vi "Get Date Yields.vi"(8 "error in (no error)":errorcluster, 11 "Programing Logic in":refnum<class "Programing Logic.lvclass">) -> (0 "error out":errorcluster, 2 "Cluster":T1, 3 "Programing Logic out":refnum<class "Programing Logic.lvclass">)   [LabVIEW 2014, in "Programing Logic.lvclass"]
uses:
  Programming Logic/Programing Logic.lvclass
  Programming Logic/Programing Logic.lvclass/Programing Logic.ctl
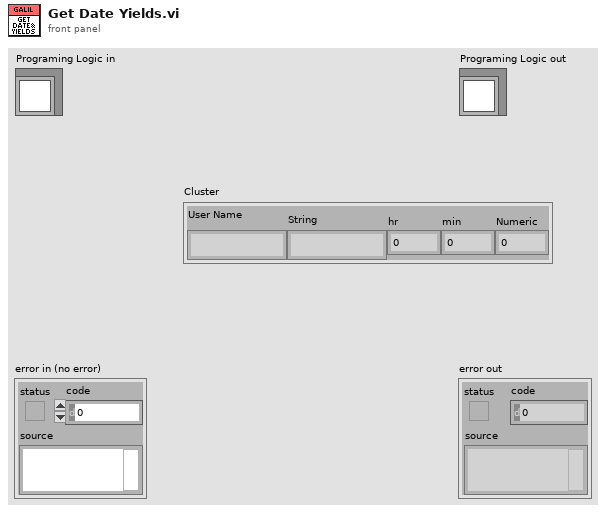
[diagram p1: front panel]
types:
  T1 = cluster{"User Name":string, "String":string, "Numeric":dbl, "min":dbl, "hr":dbl}
  T2 = cluster{"User":string, "Date":string, "Yield Counts":dbl, "minute":i32, "hour":i32}
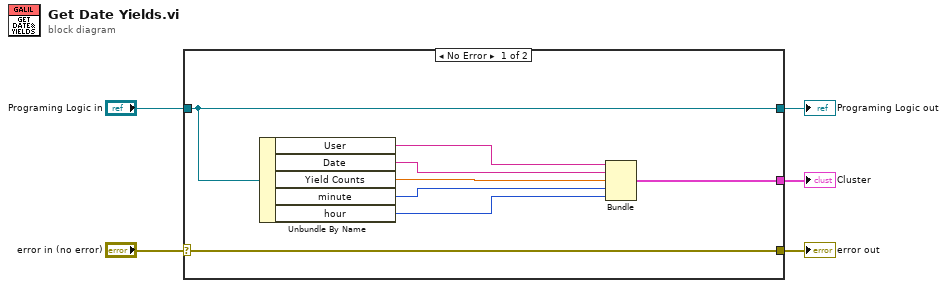
[diagram p0: block diagram]
diagram:
  n1 = case shown="No Error" "error in (no error)" {
    selector: "error in (no error)" -> [w13 w15]
    tunnel: [w13 w15] -> w4
    tunnel: [w12 w14] -> w2
    tunnel: "Programing Logic in" -> [w12 w14]
    tunnel: [w11 _] -> w1
    frame No Error {
      n2 = Unbundle By Name(w12) -> ("User"=w10:string, "Date"=w9:string, "Yield Counts"=w8:dbl, "minute"=w7:i32, "hour"=w6:i32)
      n3 = Bundle("User"=w10, "Date"=w9, "Yield Counts"=w8, "minute"=w7, "hour"=w6) -> (w11:T2)  [unwired: 1 in]
    }
    frame Error {
    }
  }
  "error out" <- w4
  "Programing Logic out" <- w2
  "Cluster" <- w1
